vi "RectangularROIonMatchPOS (SubVI).vi"(10 "Matches (pixel)":T1(array[cluster]), 11 "ROI Descriptor before matches":T3={"Global Rectangle"=[675, 567, 1751, 1642], "Contours"=[{"ID"=enum."External", "Type"=12, "Coordinates"=[1212, 1104, 85, 537, 0, 0]}]} {"Contours"."Type" items=["No Selection", "Point", "Line", "Rectangle", "Oval", "Polygon", "Freehand Region", "Annulus", "Unused2", "Unused3", "Broken Line", "Freehand Line", "Rotated Rectangle"]}) -> (2 "Array 2":dbl[](array[numeric]), 3 "ROI Descriptor after matches":T2)   [LabVIEW 2016]
panel:
  out "Bounding Box[3]":cluster{"x":sgl, "y":sgl}
  out "Bounding Box[1]":cluster{"x":sgl, "y":sgl}
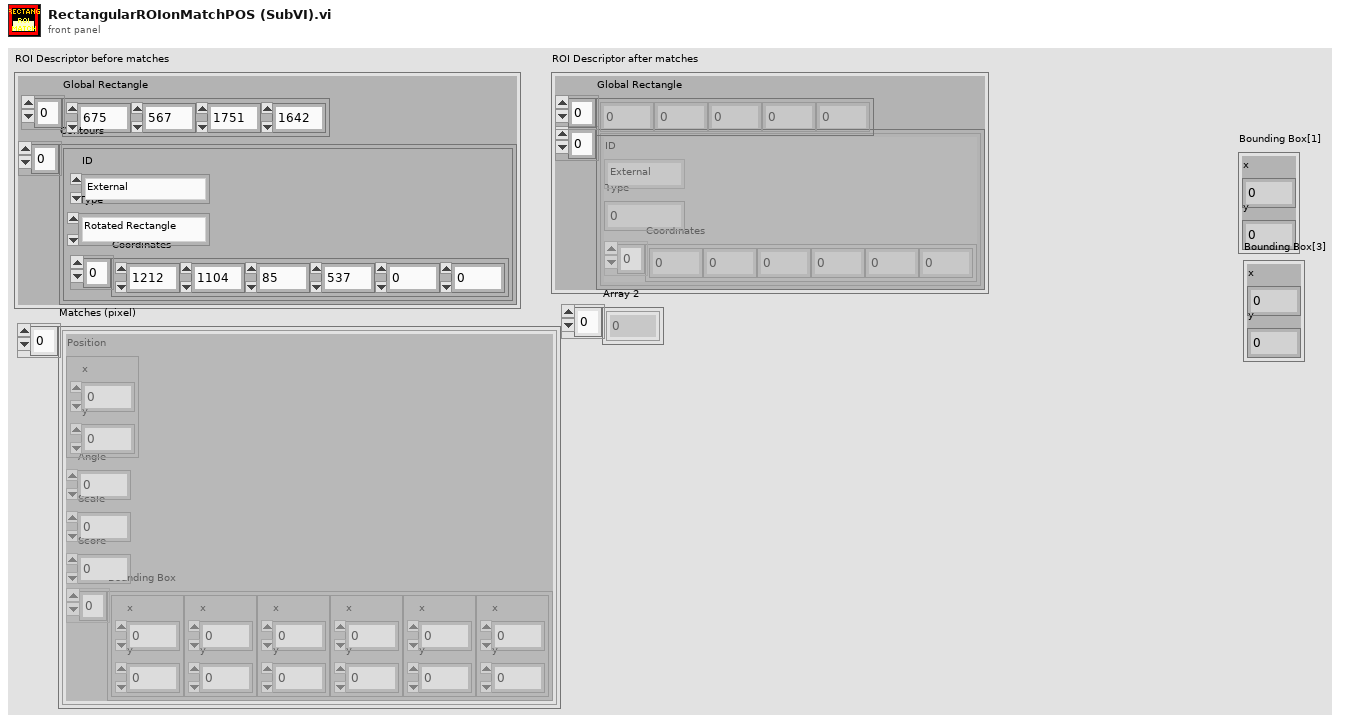
[diagram p1: front panel]
types:
  T1 = cluster{"Position":cluster{"x":sgl, "y":sgl}, "Angle":sgl, "Scale":sgl, "Score":sgl, "Bounding Box":cluster{"x":sgl, "y":sgl}[]}[]
  T2 = cluster{"Global Rectangle":i32[], cluster{"ID":enum32{"External", "Internal"}, "Type":u32, "Coordinates":i32[]}[]}
  T3 = cluster{"Global Rectangle":i32[], "Contours":cluster{"ID":enum32{"External", "Internal"}, "Type":u32, "Coordinates":i32[]}[]}
  T4 = cluster{"ID":enum32{"External", "Internal"}, "Type":u32, "Coordinates":i32[]}[]
  T5 = cluster{"Bounding Box[0]":cluster{"x":sgl, "y":sgl}, "Bounding Box[1]":cluster{"x":sgl, "y":sgl}, "Bounding Box[2]":cluster{"x":sgl, "y":sgl}, "Bounding Box[3]":cluster{"x":sgl, "y":sgl}, "Bounding Box[4]":cluster{"x":sgl, "y":sgl}, "Bounding Box[5]":cluster{"x":sgl, "y":sgl}, "Bounding Box[6]":cluster{"x":sgl, "y":sgl}, "Bounding Box[7]":cluster{"x":sgl, "y":sgl}, "Bounding Box[8]":cluster{"x":sgl, "y":sgl}}
  T6 = cluster{"ID":enum32{"External", "Internal"}, "Type":u32, "Coordinates":i32[]}
  T7 = cluster{"Coordinates":i32[], cluster{"ID":enum32{"External", "Internal"}, "Type":u32, "Coordinates":i32[]}[]}
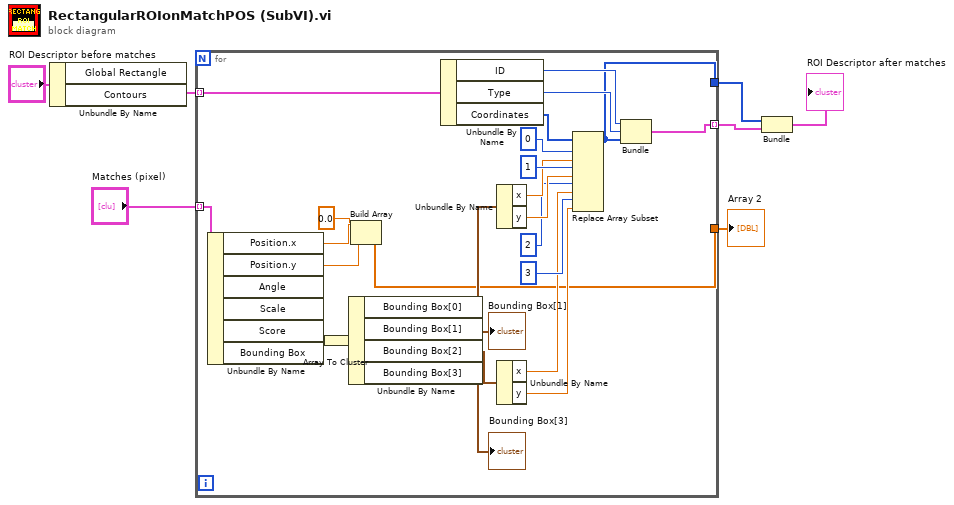
[diagram p0: block diagram]
diagram:
  n1 = Unbundle By Name("ROI Descriptor before matches") -> ("Contours"=w5:T4)  [unwired: 1 out]
  n2 = for {
    tunnel: w5 -> [w32] mode=indexing
    tunnel: "Matches (pixel)" -> [w28] mode=indexing
    tunnel: [w25] -> w7 mode=indexing
    tunnel: [w12] -> w3
    tunnel: [w9] -> w1
    n3 = Unbundle By Name(w28) -> ("Position.x"=w11:sgl, "Position.y"=w10:sgl, "Bounding Box"=w24:cluster{"x":sgl, "y":sgl}[])  [unwired: 3 out]
    n4 = Array To Cluster(array=w24) -> (cluster=w23:T5)
    n5 = Unbundle By Name(w23) -> ("Bounding Box[0]"=w20:cluster{"x":sgl, "y":sgl}, "Bounding Box[1]"=→"Bounding Box[1]":cluster{"x":sgl, "y":sgl}, "Bounding Box[2]"=w15:cluster{"x":sgl, "y":sgl}, "Bounding Box[3]"=→"Bounding Box[3]":cluster{"x":sgl, "y":sgl})
    n6 = Build Array(w11, w10, 0.0 ("element")) -> (w9:dbl[])
    n7 = Unbundle By Name(w32) -> ("ID"=w26:enum32{"External", "Internal"}, "Type"=w27:u32, "Coordinates"=w31:i32[])
    n8 = Unbundle By Name(w20) -> ("x"=w19:sgl, "y"=w18:sgl)
    n9 = Unbundle By Name(w15) -> ("x"=w14:sgl, "y"=w13:sgl)
    n10 = Replace Array Subset(array=w31, new element #1=w19, index #1=0 ("index"), new element #2=w18, index #2=1 ("index"), new element #3=w14, index #3=2 ("index"), new element #4=w13, index #4=3 ("index")) -> (w12:i32[])
    n11 = Bundle("ID"=w26, "Type"=w27, "Coordinates"=w12) -> (w25:T6)  [unwired: 1 in]
  }
  "Array 2" <- w1
  n12 = Bundle("Coordinates"=w3, w7) -> (→"ROI Descriptor after matches":T7)  [unwired: 1 in]
